vi "m1m3_getEvent_PIDInfo.vi"(8 "error in (no error)":errorcluster, 11 "logevent_PIDInfo_Ctl":T1={"Timestamp"=0.0, "Timestep[6]"=[0.0, 0.0, 0.0, 0.0, 0.0, 0.0], "P[6]"=[0.0, 0.0, 0.0, 0.0, 0.0, 0.0], "I[6]"=[0.0, 0.0, 0.0, 0.0, 0.0, 0.0], "D[6]"=[0.0, 0.0, 0.0, 0.0, 0.0, 0.0], "N[6]"=[0.0, 0.0, 0.0, 0.0, 0.0, 0.0], "CalculatedA[6]"=[0.0, 0.0, 0.0, 0.0, 0.0, 0.0], "CalculatedB[6]"=[0.0, 0.0, 0.0, 0.0, 0.0, 0.0], "CalculatedC[6]"=[0.0, 0.0, 0.0, 0.0, 0.0, 0.0], "CalculatedD[6]"=[0.0, 0.0, 0.0, 0.0, 0.0, 0.0], "CalculatedE[6]"=[0.0, 0.0, 0.0, 0.0, 0.0, 0.0], "priority"=0}) -> (0 "error out":errorcluster, 2 "function return":i32, 3 "logevent_PIDInfo_Ctl out":T1)   [LabVIEW 2016, in "SALLV_m1m3.lvlib"]
doc: "int m1m3_shm_getEvent_PIDInfoLV(m1m3_logevent_PIDInfoLV *logevent_PIDInfo_Ctl );"
uses:
  SALLV_m1m3.lvlib
  DataTypes/logevent_PIDInfo.ctl
  SALLV_m1m3.so
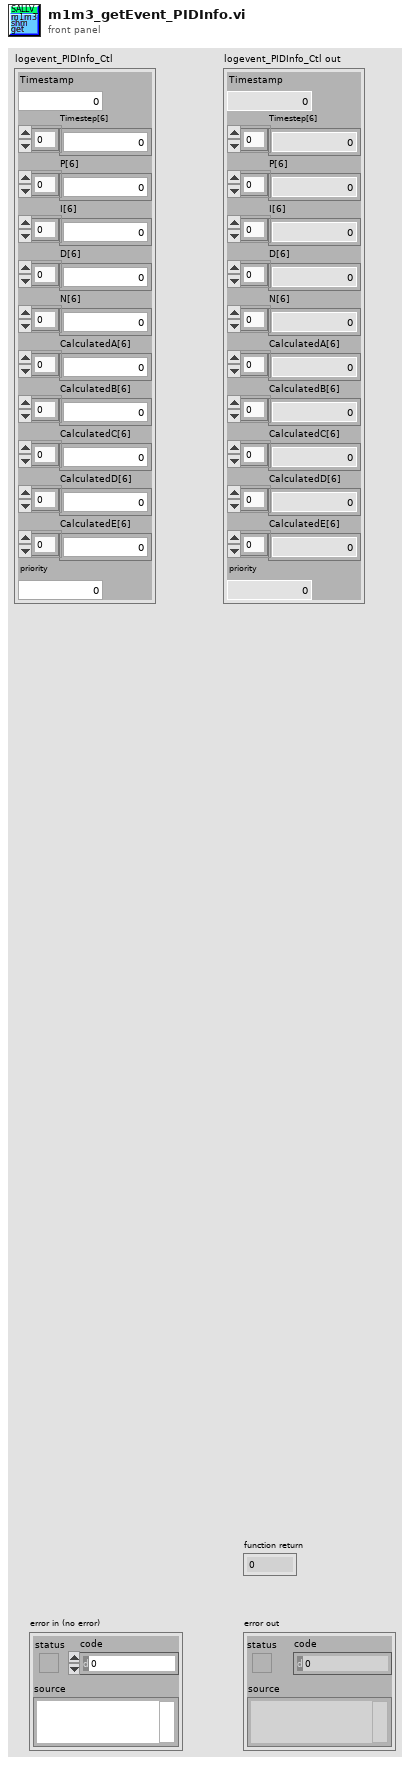
[diagram p1: front panel]
types:
  T1 = typedef "SALLV_m1m3.lvlib/logevent_PIDInfo.ctl" = cluster{"Timestamp":dbl, "Timestep[6]":dbl[], "P[6]":dbl[], "I[6]":dbl[], "D[6]":dbl[], "N[6]":dbl[], "CalculatedA[6]":dbl[], "CalculatedB[6]":dbl[], "CalculatedC[6]":dbl[], "CalculatedD[6]":dbl[], "CalculatedE[6]":dbl[], "priority":i32}
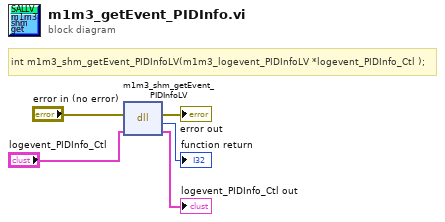
[diagram p0: block diagram]
diagram:
  # "int m1m3_shm_getEvent_PIDInfoLV(m1m3_logevent_PIDInfoLV *logevent_PIDInfo_Ctl );"
  n1 = dll-call lib="opt/CODE/SALLV_m1m3/SALLV_m1m3.*" fn="m1m3_shm_getEvent_PIDInfoLV"(error in="error in (no error)", "logevent_PIDInfo_Ctl"="logevent_PIDInfo_Ctl") -> (error out=→"error out":errorcluster, →"function return":i32, "logevent_PIDInfo_Ctl"=→"logevent_PIDInfo_Ctl out":T1)  [unwired: 2 in, 1 out]
